vi "Init Power.vi"(8 "error in":errorcluster, 11 "Controller in":refnum<class "Controller.lvclass">) -> (0 "error out":errorcluster, 3 "Controller out":refnum<class "Controller.lvclass">)   [LabVIEW 2014, in "Controller.lvlib" / "Controller.lvclass"]
uses:
  Controller.lvclass
  Messages/Power Supply/PowerSupply MSG.lvclass
  <vilib>/ActorFramework/Actor/Actor.lvclass/Actor.ctl
  <vilib>/ActorFramework/Message Enqueuer/Message Enqueuer.lvclass/Message Enqueuer.ctl
  Messages/Power Supply/PowerSupply MSG.lvclass/PowerSupply MSG.ctl
  Messages/Power Supply/Write Value.vi
  <vilib>/ActorFramework/Message Enqueuer/Init from Existing Queue.vi
  <vilib>/Utility/config.llb/Read Key (Boolean).vi
  <vilib>/ActorFramework/Message Priority Queue/Priority Enqueue.vi
  <vilib>/ActorFramework/Message Enqueuer/Message Enqueuer.lvclass
  <vilib>/Utility/config.llb/NI_LVConfig.lvlib
  <vilib>/ActorFramework/Actor/Actor.lvclass
  SuperActor/Ex Nested.lvclass
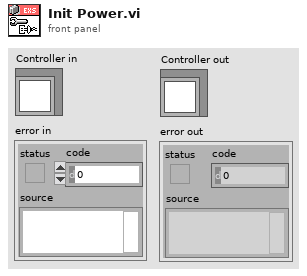
[diagram p1: front panel]
types:
  T1 = typedef "NI_LVConfig.lvlib/Config Data RefNum.ctl" = refnum<k1>
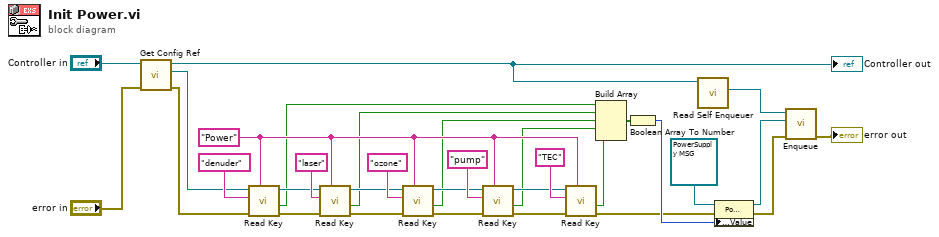
[diagram p0: block diagram]
diagram:
  w23 = "Power" ("section")
  n1 = call "Get Config Ref.vi"("error in"="error in", "Ex Nested in"="Controller in") -> ("error out"=w4:errorcluster, "config ref"=w3:T1, "Ex Nested out"=w1:refnum<class "Controller.lvclass">)  [unwired: 7 in]
  "Controller out" <- w1
  n2 = call-poly <vilib>:"Read Key.vi"("section"=w23, "error in (no error)"=w4, "key"="denuder", "refnum"=w3) -> ("error out"=w17:errorcluster, "value"=w22:bool, "refnum out"=w30:T1)  [unwired: 4 in, 1 out]
  n3 = call-poly <vilib>:"Read Key.vi"("section"=w23, "error in (no error)"=w17, "key"="laser", "refnum"=w30) -> ("error out"=w16:errorcluster, "value"=w21:bool, "refnum out"=w28:T1)  [unwired: 4 in, 1 out]
  n4 = call-poly <vilib>:"Read Key.vi"("section"=w23, "error in (no error)"=w16, "key"="ozone", "refnum"=w28) -> ("error out"=w15:errorcluster, "value"=w20:bool, "refnum out"=w26:T1)  [unwired: 4 in, 1 out]
  n5 = call-poly <vilib>:"Read Key.vi"("section"=w23, "error in (no error)"=w15, "key"="pump", "refnum"=w26) -> ("error out"=w14:errorcluster, "value"=w19:bool, "refnum out"=w24:T1)  [unwired: 4 in, 1 out]
  n6 = call-poly <vilib>:"Read Key.vi"("section"=w23, "error in (no error)"=w14, "key"="TEC", "refnum"=w24) -> ("error out"=w8:errorcluster, "value"=w18:bool)  [unwired: 4 in, 2 out]
  n7 = Build Array(w22, w21, w20, w19, w18) -> (w12:bool[])
  n8 = Boolean Array To Number(Boolean array=w12) -> (number=w10:u32)
  n9 = call <vilib>:"Read Self Enqueuer.vi"("Actor"=w1) -> ("Self Enqueuer"=w13:refnum<class "Message Enqueuer.lvclass">)  [unwired: 10 in]
  n10 = property class="PowerSupply MSG"(reference=refnum<class "PowerSupply MSG.lvclass"> refnum ("Controller.lvlib:PowerSupply MSG"), error in=w8, "Accessors:Value"=w10) -> (reference out=w9:refnum<class "PowerSupply MSG.lvclass">, error out=w7:errorcluster)
  n11 = call <vilib>:"Enqueue.vi"("error in (no error)"=w7, "Message"=w9, "Message Enqueuer in"=w13) -> ("error out"=→"error out":errorcluster)  [unwired: 7 in, 1 out]
